vi "let.vi"() -> ()   [LabVIEW 2017]
uses:
  <vilib>/LVH/i3 JSON/JSON Generation/Create Value Files/Create Value - Object.vi
  <vilib>/LVH/i3 JSON/JSON Generation/Add Object Parameter Files/Add Object Parameter - String.vi
  <vilib>/LVH/i3 JSON/JSON Parsing/Get Object Parameter Files/Get Object Parameter - String.vi
  <vilib>/LVH/i3 JSON/i3-json.lvlib
  <vilib>/LVH/i3 JSON/JSON Generation/Add Object Parameter Files/Add Object Parameter - Object.vi
panel:
  out "JSON Tree Out Passthrough":variant
  out "String Value":string
  out "String":string
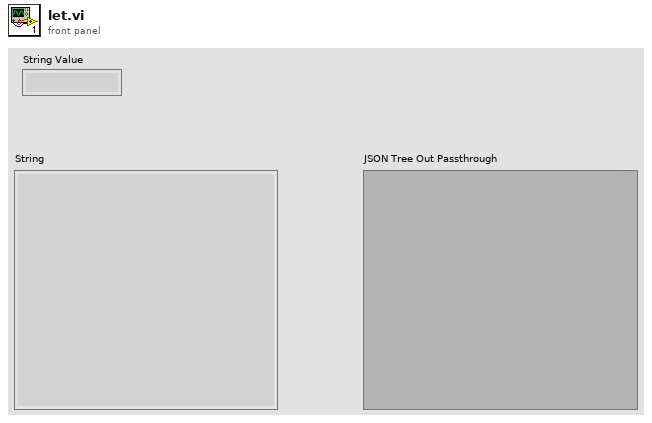
[diagram p1: front panel]
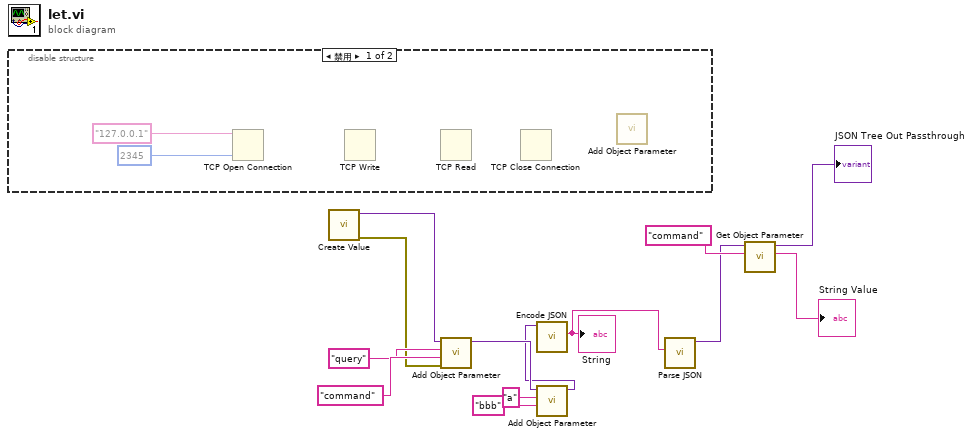
[diagram p0: block diagram]
diagram:
  n1 = disable-structure shown="禁用" {
    frame Disabled {
      n2 = TCP Open Connection(address="127.0.0.1" ("地址"), remote port or service name=u16 2345 ("远程端口或服务名称")) -> ()  [unwired: 3 in, 2 out]
      n3 = TCP Write() -> ()  [unwired: 4 in, 3 out]
      n4 = TCP Read() -> ()  [unwired: 5 in, 3 out]
      n5 = TCP Close Connection() -> ()  [unwired: 3 in, 2 out]
      n6 = call-poly <vilib>:"Add Object Parameter.vi"() -> ()  [unwired: 10 in, 2 out]
    }
    frame Enabled {
    }
  }
  n7 = call-poly <vilib>:"Create Value.vi"() -> ("error out"=w10:errorcluster, "JSON Tree"=w11:variant)  [unwired: 10 in]
  n8 = call-poly <vilib>:"Add Object Parameter.vi"("error in (no error)"=w10, "Name"="command", "String"="query", "JSON Tree in (JSON Object)"=w11) -> ("JSON Tree out (JSON Object)"=w6:variant)  [unwired: 6 in, 1 out]
  n9 = call-poly <vilib>:"Add Object Parameter.vi"("Name"="bbb", "String"="a", "JSON Tree in (JSON Object)"=w6) -> ("JSON Tree out (JSON Object)"=w5:variant)  [unwired: 7 in, 1 out]
  n10 = call <vilib>:"Encode JSON.vi"("JSON Tree"=w5) -> ("String"=w9:string)  [unwired: 5 in, 1 out]
  "String" <- w9
  n11 = call <vilib>:"Parse JSON.vi"("JSON String"=w9) -> ("JSON Tree"=w2:variant)  [unwired: 7 in, 3 out]
  n12 = call-poly <vilib>:"Get Object Parameter.vi"("Parameter Name"="command", "JSON Tree In (JSON Object)"=w2) -> ("String Value"=→"String Value":string, "JSON Tree Out Passthrough"=→"JSON Tree Out Passthrough":variant)  [unwired: 6 in, 2 out]
